vi "Pack Bits (SubVI).vi"(0 "Input Valid?":bool, 2 "Data In":u8, 5 "Bit Depth":u8) -> (14 "Output Valid?":bool, 19 "Data Out":u8)   [LabVIEW 2014]
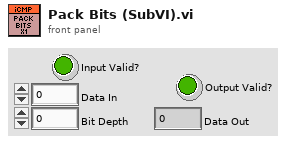
[diagram p1: front panel]
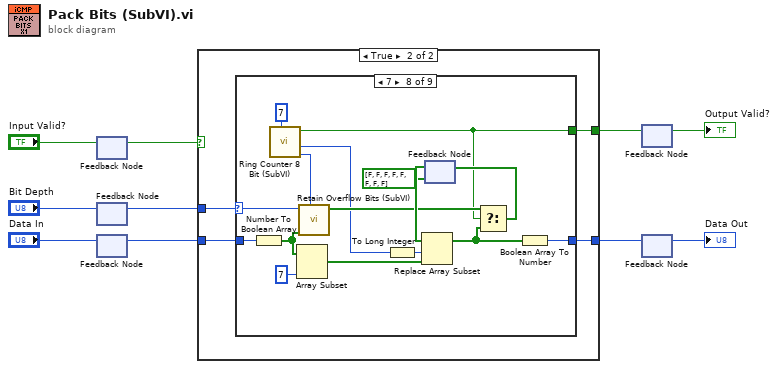
[diagram p0: block diagram]
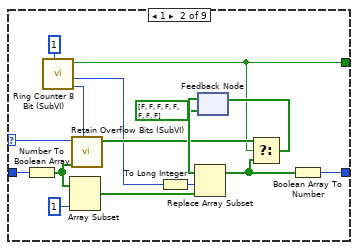
[diagram p4: hidden frame]
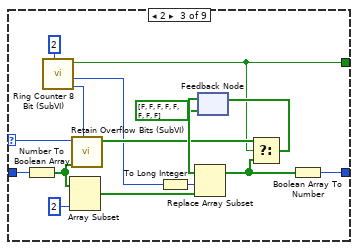
[diagram p5: hidden frame]
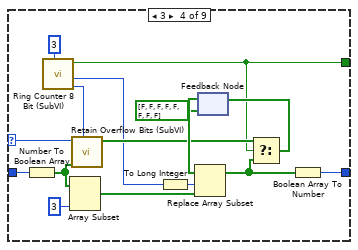
[diagram p6: hidden frame]
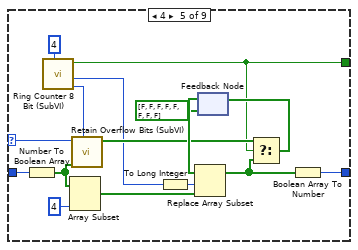
[diagram p7: hidden frame]
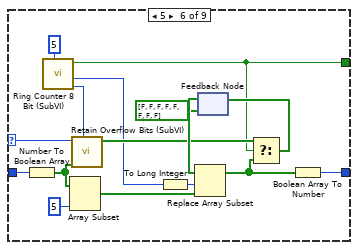
[diagram p8: hidden frame]
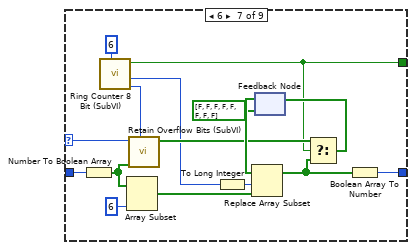
[diagram p9: hidden frame]
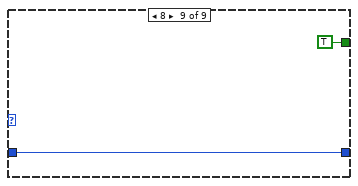
[diagram p10: hidden frame]
diagram:
  n1 = feedback-in #1("Input Valid?") -> ()
  n2 = feedback #1() -> (w5:bool)  [unwired: 1 in]
  n3 = feedback-in #2("Bit Depth") -> ()
  n4 = feedback #2() -> (w4:u8)  [unwired: 1 in]
  n5 = feedback-in #3("Data In") -> ()
  n6 = feedback #3() -> (w3:u8)  [unwired: 1 in]
  n7 = case shown="True" w5 {
    tunnel: [_ w14] -> w6
    tunnel: [_ w13] -> w7
    tunnel: w3 -> [_ w12]
    tunnel: w4 -> [_ w11]
    frame False {
    }
    frame True {
      n8 = case shown="7" w11 {
        selector: w11 -> [_ w16 w32 w48 w64 w79 w96 w112 _]
        tunnel: [_ w19 w35 w51 w67 w83 w99 w115 TRUE ("End of Count?")] -> w13
        tunnel: w12 -> [_ w30 w46 w62 w78 w94 w110 w126 w128]
        tunnel: [_ w26 w42 w58 w74 w90 w106 w122 w128] -> w14
        frame 0, Default {
        }
        frame 1 {
          n9 = Number To Boolean Array(number=w30) -> (Boolean array=w15:bool[])
          n10 = call "Ring Counter 8 Bit (SubVI).vi"("Increment"=u8 1) -> ("Next Count"=w18:u8, "Count"=w17:u8, "End of Count?"=w19:bool)  [unwired: 8 in]
          n11 = Array Subset(array=w15, length=1) -> (w23:bool[])  [unwired: 1 in]
          n12 = call "Retain Overflow Bits (SubVI).vi"("N Overflow Bits"=w18, "Bit Array In"=w15, "Bit Depth"=w16) -> ("Bit Array Out"=w21:bool[])  [unwired: 8 in]
          n13 = To Long Integer(number=w17) -> (32bit integer=w28:i32)
          n14 = feedback #4(bool[] [FALSE, FALSE, FALSE, FALSE, FALSE, FALSE, FALSE, FALSE]) -> (w27:bool[])
          n15 = Replace Array Subset(array=w27, new element=w23, index=w28) -> (w25:bool[])
          n16 = Select(t=w21, s=w19, f=w25) -> (s? t:f=w24:bool[])
          n17 = feedback-in #4(w24) -> ()
          n18 = Boolean Array To Number(Boolean array=w25) -> (number=w26:u8)
        }
        frame 2 {
          n19 = Number To Boolean Array(number=w46) -> (Boolean array=w31:bool[])
          n20 = call "Ring Counter 8 Bit (SubVI).vi"("Increment"=u8 2) -> ("Next Count"=w34:u8, "Count"=w33:u8, "End of Count?"=w35:bool)  [unwired: 8 in]
          n21 = Array Subset(array=w31, length=2) -> (w39:bool[])  [unwired: 1 in]
          n22 = call "Retain Overflow Bits (SubVI).vi"("N Overflow Bits"=w34, "Bit Array In"=w31, "Bit Depth"=w32) -> ("Bit Array Out"=w37:bool[])  [unwired: 8 in]
          n23 = To Long Integer(number=w33) -> (32bit integer=w44:i32)
          n24 = feedback #5(bool[] [FALSE, FALSE, FALSE, FALSE, FALSE, FALSE, FALSE, FALSE]) -> (w43:bool[])
          n25 = Replace Array Subset(array=w43, new element=w39, index=w44) -> (w41:bool[])
          n26 = Select(t=w37, s=w35, f=w41) -> (s? t:f=w40:bool[])
          n27 = feedback-in #5(w40) -> ()
          n28 = Boolean Array To Number(Boolean array=w41) -> (number=w42:u8)
        }
        frame 3 {
          n29 = Number To Boolean Array(number=w62) -> (Boolean array=w47:bool[])
          n30 = call "Ring Counter 8 Bit (SubVI).vi"("Increment"=u8 3) -> ("Next Count"=w50:u8, "Count"=w49:u8, "End of Count?"=w51:bool)  [unwired: 8 in]
          n31 = Array Subset(array=w47, length=3) -> (w55:bool[])  [unwired: 1 in]
          n32 = call "Retain Overflow Bits (SubVI).vi"("N Overflow Bits"=w50, "Bit Array In"=w47, "Bit Depth"=w48) -> ("Bit Array Out"=w53:bool[])  [unwired: 8 in]
          n33 = To Long Integer(number=w49) -> (32bit integer=w60:i32)
          n34 = feedback #6(bool[] [FALSE, FALSE, FALSE, FALSE, FALSE, FALSE, FALSE, FALSE]) -> (w59:bool[])
          n35 = Replace Array Subset(array=w59, new element=w55, index=w60) -> (w57:bool[])
          n36 = Select(t=w53, s=w51, f=w57) -> (s? t:f=w56:bool[])
          n37 = feedback-in #6(w56) -> ()
          n38 = Boolean Array To Number(Boolean array=w57) -> (number=w58:u8)
        }
        frame 4 {
          n39 = Number To Boolean Array(number=w78) -> (Boolean array=w63:bool[])
          n40 = call "Ring Counter 8 Bit (SubVI).vi"("Increment"=u8 4) -> ("Next Count"=w66:u8, "Count"=w65:u8, "End of Count?"=w67:bool)  [unwired: 8 in]
          n41 = Array Subset(array=w63, length=4) -> (w71:bool[])  [unwired: 1 in]
          n42 = call "Retain Overflow Bits (SubVI).vi"("N Overflow Bits"=w66, "Bit Array In"=w63, "Bit Depth"=w64) -> ("Bit Array Out"=w69:bool[])  [unwired: 8 in]
          n43 = To Long Integer(number=w65) -> (32bit integer=w76:i32)
          n44 = feedback #7(bool[] [FALSE, FALSE, FALSE, FALSE, FALSE, FALSE, FALSE, FALSE]) -> (w75:bool[])
          n45 = Replace Array Subset(array=w75, new element=w71, index=w76) -> (w73:bool[])
          n46 = Select(t=w69, s=w67, f=w73) -> (s? t:f=w72:bool[])
          n47 = feedback-in #7(w72) -> ()
          n48 = Boolean Array To Number(Boolean array=w73) -> (number=w74:u8)
        }
        frame 5 {
          n49 = Number To Boolean Array(number=w94) -> (Boolean array=w80:bool[])
          n50 = call "Ring Counter 8 Bit (SubVI).vi"("Increment"=u8 5) -> ("Next Count"=w82:u8, "Count"=w81:u8, "End of Count?"=w83:bool)  [unwired: 8 in]
          n51 = Array Subset(array=w80, length=5) -> (w87:bool[])  [unwired: 1 in]
          n52 = call "Retain Overflow Bits (SubVI).vi"("N Overflow Bits"=w82, "Bit Array In"=w80, "Bit Depth"=w79) -> ("Bit Array Out"=w85:bool[])  [unwired: 8 in]
          n53 = To Long Integer(number=w81) -> (32bit integer=w92:i32)
          n54 = feedback #8(bool[] [FALSE, FALSE, FALSE, FALSE, FALSE, FALSE, FALSE, FALSE]) -> (w91:bool[])
          n55 = Replace Array Subset(array=w91, new element=w87, index=w92) -> (w89:bool[])
          n56 = Select(t=w85, s=w83, f=w89) -> (s? t:f=w88:bool[])
          n57 = feedback-in #8(w88) -> ()
          n58 = Boolean Array To Number(Boolean array=w89) -> (number=w90:u8)
        }
        frame 6 {
          n59 = Number To Boolean Array(number=w110) -> (Boolean array=w95:bool[])
          n60 = call "Ring Counter 8 Bit (SubVI).vi"("Increment"=u8 6) -> ("Next Count"=w98:u8, "Count"=w97:u8, "End of Count?"=w99:bool)  [unwired: 8 in]
          n61 = Array Subset(array=w95, length=6) -> (w103:bool[])  [unwired: 1 in]
          n62 = call "Retain Overflow Bits (SubVI).vi"("N Overflow Bits"=w98, "Bit Array In"=w95, "Bit Depth"=w96) -> ("Bit Array Out"=w101:bool[])  [unwired: 8 in]
          n63 = To Long Integer(number=w97) -> (32bit integer=w108:i32)
          n64 = feedback #9(bool[] [FALSE, FALSE, FALSE, FALSE, FALSE, FALSE, FALSE, FALSE]) -> (w107:bool[])
          n65 = Replace Array Subset(array=w107, new element=w103, index=w108) -> (w105:bool[])
          n66 = Select(t=w101, s=w99, f=w105) -> (s? t:f=w104:bool[])
          n67 = feedback-in #9(w104) -> ()
          n68 = Boolean Array To Number(Boolean array=w105) -> (number=w106:u8)
        }
        frame 7 {
          n69 = Number To Boolean Array(number=w126) -> (Boolean array=w111:bool[])
          n70 = call "Ring Counter 8 Bit (SubVI).vi"("Increment"=u8 7) -> ("Next Count"=w114:u8, "Count"=w113:u8, "End of Count?"=w115:bool)  [unwired: 8 in]
          n71 = Array Subset(array=w111, length=7) -> (w119:bool[])  [unwired: 1 in]
          n72 = call "Retain Overflow Bits (SubVI).vi"("N Overflow Bits"=w114, "Bit Array In"=w111, "Bit Depth"=w112) -> ("Bit Array Out"=w117:bool[])  [unwired: 8 in]
          n73 = To Long Integer(number=w113) -> (32bit integer=w124:i32)
          n74 = feedback #10(bool[] [FALSE, FALSE, FALSE, FALSE, FALSE, FALSE, FALSE, FALSE]) -> (w123:bool[])
          n75 = Replace Array Subset(array=w123, new element=w119, index=w124) -> (w121:bool[])
          n76 = Select(t=w117, s=w115, f=w121) -> (s? t:f=w120:bool[])
          n77 = feedback-in #10(w120) -> ()
          n78 = Boolean Array To Number(Boolean array=w121) -> (number=w122:u8)
        }
        frame 8 {
        }
      }
    }
  }
  n79 = feedback-in #11(w7) -> ()
  n80 = feedback #11() -> (→"Output Valid?":bool)  [unwired: 1 in]
  n81 = feedback-in #12(w6) -> ()
  n82 = feedback #12() -> (→"Data Out":u8)  [unwired: 1 in]
